vi "Read Instrument.DAQ.vi"(8 "error in (no error)":errorcluster, 11 "Instrument.Lockin in":refnum<class "Instrument.Lockin.lvclass">) -> (0 "error out":errorcluster, 2 "Instrument.DAQ":refnum<class "Instrument.DAQ.lvclass">, 3 "Instrument.Lockin out":refnum<class "Instrument.Lockin.lvclass">)   [LabVIEW 2019, in "Instrument.Lockin.lvclass"]
uses:
  Instrument.Lockin.lvclass
  C:/Program Files (x86)/National Instruments/LabVIEW 2019/vi.lib/JKI/JKI SMO/SMO/SMO.lvclass
  Instrument.DAQ/Instrument.DAQ.lvclass
  Instrument.Lockin.lvclass/Instrument.Lockin.ctl
  <vilib>/JKI/JKI SMO/SMO/SMO.lvclass
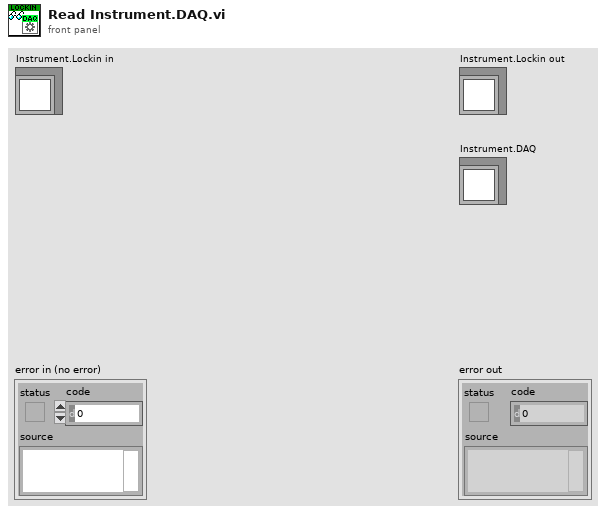
[diagram p1: front panel]
types:
  T1 = typedef "Instrument.Lockin.lvclass/Lockin.Dependencies--Cluster.ctl" = cluster{"Instrument.DAQ":refnum<class "Instrument.DAQ.lvclass">}
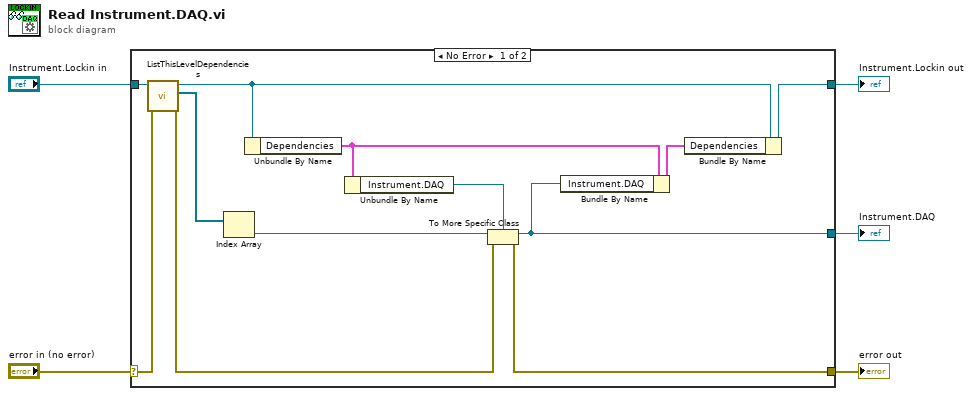
[diagram p0: block diagram]
diagram:
  n1 = case shown="No Error" "error in (no error)" {
    selector: "error in (no error)" -> [w13 w18]
    tunnel: [w9 w18] -> w4
    tunnel: [w6 w19] -> w2
    tunnel: "Instrument.Lockin in" -> [w11 w19]
    tunnel: [w8 _] -> w1
    frame No Error {
      n2 = call <vilib>:"ListThisLevelDependencies.vi"("error in (no error)"=w13, "SMO in"=w11) -> ("error out"=w10:errorcluster, "[My Dependencies]"=w15:refnum<class "SMO.lvclass">[], "SMO out"=w7:refnum<class "Instrument.Lockin.lvclass">)  [unwired: 7 in]
      n3 = Index Array(array=w15) -> (element=w12:refnum<class "SMO.lvclass">)  [unwired: 1 in]
      n4 = Unbundle By Name(w7) -> ("Dependencies"=w16:T1)
      n5 = Unbundle By Name(w16) -> ("Instrument.DAQ"=w17:refnum<class "Instrument.DAQ.lvclass">)
      n6 = To More Specific Class(target class=w17, reference=w12, error in=w10) -> (specific class reference=w8:refnum<class "Instrument.DAQ.lvclass">, error out=w9:errorcluster)
      n7 = Bundle By Name(cluster=w16, "Instrument.DAQ"=w8) -> (w14:T1)
      n8 = Bundle By Name(cluster=w7, "Dependencies"=w14) -> (w6:refnum<class "Instrument.Lockin.lvclass">)
    }
    frame Error {
    }
  }
  "error out" <- w4
  "Instrument.Lockin out" <- w2
  "Instrument.DAQ" <- w1
